vi "Read Message Type and Terminals.vi"(8 "error in":errorcluster, 11 "message ref in":refnum<k20>) -> (0 "error out":errorcluster, 2 "message type":T3, 3 "message ref out":refnum<k20>, 4 "Rx terminal":T1, 6 "Tx terminal":T1)   [LabVIEW 2020, in "MIL-STD 1553 Import.lvlib"]
uses:
  MIL-STD 1553 Import.lvlib
  Shared/Message Type.ctl
  Shared/Terminal Endpoint.ctl
  Shared/Address.ctl
  40e07135-e19e-4b22-895a-2c183958625d.vi
  487ea7c7-ffca-4428-88f2-a900c8ae7e8d.vi
  40e07135-e19e-4b22-895a-2c183958625d.vi/b1e6fcf8-dac1-42d2-b1fe-151afe06dbd4.vi
  487ea7c7-ffca-4428-88f2-a900c8ae7e8d.vi/b1e6fcf8-dac1-42d2-b1fe-151afe06dbd4.vi
  Constants.vi
  <vilib>/xml/Get Node Text Content.vi
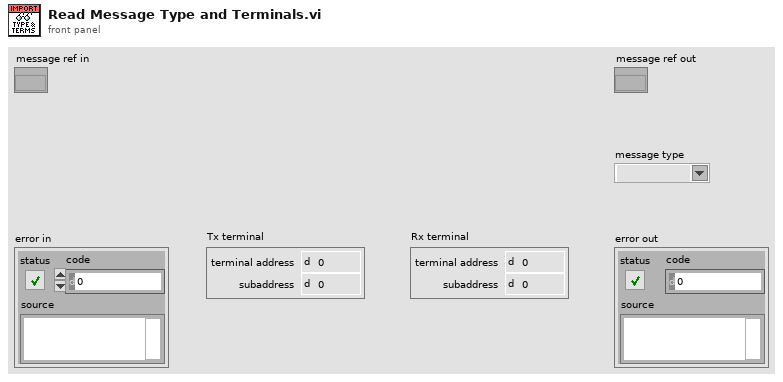
[diagram p1: front panel]
types:
  T1 = typedef "Terminal Endpoint.ctl" = cluster{"terminal address":T2, "subaddress":T2}
  T2 = typedef "Address.ctl" = u16
  T3 = typedef "Message Type.ctl" = string
  T4 = cluster{"terminal address":bool, "subaddress":bool}
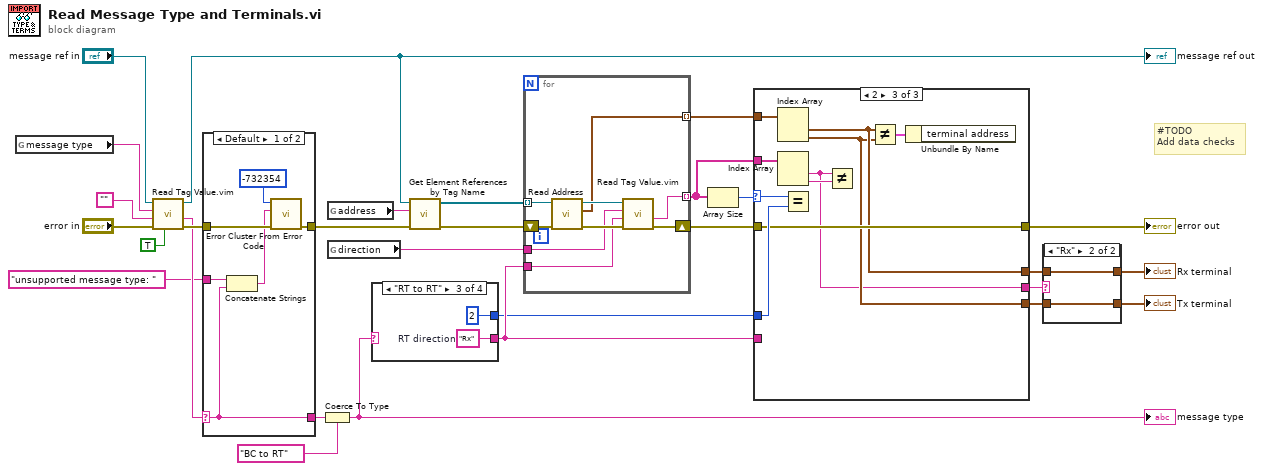
[diagram p0: block diagram]
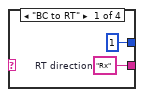
[diagram p3: hidden frame]
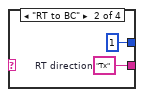
[diagram p4: hidden frame]
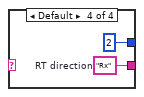
[diagram p5: hidden frame]
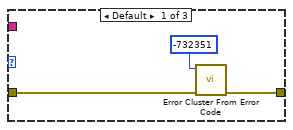
[diagram p6: hidden frame]
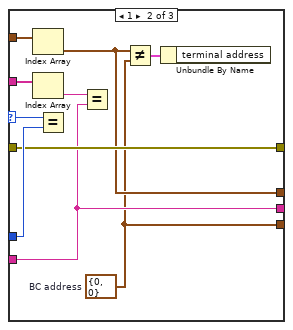
[diagram p7: hidden frame]
diagram:
  # "#TODO\nAdd data checks"
  n1 = global read "Constants.vi" "message type"() -> (w29:string)
  n2 = call "Read Tag Value.vim"("required (F)"=TRUE, "error in"="error in", "default"="", "tag name"=w29, "node in"="message ref in") -> ("error out"=w23:errorcluster, "value"=w22:string, "node out"=w19:refnum<k20>)  [unwired: 4 in]
  "message ref out" <- w19
  n3 = case shown="Default" w22 {
    selector: w22 -> [w31 w36]
    tunnel: [w34 w37] -> w21
    tunnel: w23 -> [w35 w37]
    tunnel: [w31 w36] -> w25
    tunnel: "unsupported message type: " -> [w32 _]
    frame Default {
      n4 = Concatenate Strings(w32, w31) -> (w30:string)
      n5 = call <vilib>:"Error Cluster From Error Code.vi"("error in (no error)"=w35, "error message (\"\")"=w30, "error code (0)"=-732354) -> ("error out"=w34:errorcluster)  [unwired: 6 in]
    }
    frame "BC to RT", "MC", "RT to BC", "RT to RT" {
    }
  }
  n6 = Coerce To Type(0:w25, 1:T3 "BC to RT" ("message type")) -> (2:w7:T3)
  "message type" <- w7
  n7 = global read "Constants.vi" "address"() -> (w20:string)
  n8 = global read "Constants.vi" "direction"() -> (w16:string)
  n9 = case shown="\"RT to RT\"" w7 {
    tunnel: [w39 w41 w43 w45] -> w9
    tunnel: [1 1 2 2] -> w8
    frame "BC to RT" {
      w39 = "Rx"  # RT direction
    }
    frame "RT to BC" {
      w41 = "Tx"  # RT direction
    }
    frame "RT to RT" {
      w43 = "Rx"  # RT direction
    }
    frame Default {
      w45 = "Rx"  # RT direction
    }
  }
  n10 = call "Get Element References by Tag Name.vi"("error in"=w21, "tag name"=w20, "node in"=w19) -> ("error out"=w18:errorcluster, "array of elements"=w17:refnum<k20>[])  [unwired: 7 in]
  n11 = for {
    shift-right: [w52] -> w15
    shift-left: w18 -> [w54]
    tunnel: w17 -> [w51] mode=indexing
    tunnel: w16 -> [w49]
    tunnel: w9 -> [w48]
    tunnel: [w47] -> w11 mode=indexing
    tunnel: [w46] -> w10 mode=indexing
    n12 = call "Read Address.vi"("error in"=w54, "address ref in"=w51) -> ("error out"=w53:errorcluster, "terminal"=w46:T1, "address ref out"=w50:refnum<k20>)  [unwired: 7 in]
    n13 = call "Read Tag Value.vim"("error in"=w53, "default"=w48, "tag name"=w49, "node in"=w50) -> ("error out"=w52:errorcluster, "value"=w47:string)  [unwired: 5 in, 1 out]
  }
  n14 = Array Size(array=w11) -> (size(s)=w12:i32)
  n15 = case shown="2" w12 {
    selector: w12 -> [_ w63 w74]
    tunnel: w15 -> [w56 w61 w71]
    tunnel: [w55 w61 w71] -> w14
    tunnel: w11 -> [_ w67 w77]
    tunnel: w10 -> [_ w66 w76]
    tunnel: w9 -> [_ w60 _]
    tunnel: w8 -> [_ w62 w73]
    tunnel: [_ w59 w70] -> w4
    tunnel: [_ w58 w69] -> w3
    tunnel: [_ w60 w68] -> w5
    frame Default {
      n16 = call <vilib>:"Error Cluster From Error Code.vi"("error in (no error)"=w56, "error code (0)"=-732351) -> ("error out"=w55:errorcluster)  [unwired: 7 in]
    }
    frame 1 {
      w58 = T1 {"terminal address"=0, "subaddress"=0}  # BC address
      n17 = Index Array(array=w66) -> (element=w59:T1)  [unwired: 1 in]
      n18 = Index Array(array=w67) -> (element=w64:string)  [unwired: 1 in]
      n19 = Equal?(x=w63, y=w62) -> ()  [unwired: 1 out]
      n20 = Equal?(x=w64, y=w60) -> ()  [unwired: 1 out]
      n21 = Not Equal?(x=w59, y=w58) -> (x != y?=w65:T4)
      n22 = Unbundle By Name(w65) -> ()  [unwired: 1 out]
    }
    frame 2 {
      n23 = Index Array(array=w76) -> (element #1=w70:T1, element #2=w69:T1)  [unwired: 2 in]
      n24 = Index Array(array=w77) -> (element #1=w68:string, element #2=w72:string)  [unwired: 2 in]
      n25 = Equal?(x=w74, y=w73) -> ()  [unwired: 1 out]
      n26 = Not Equal?(x=w68, y=w72) -> ()  [unwired: 1 out]
      n27 = Not Equal?(x=w70, y=w69) -> (x != y?=w75:T4)
      n28 = Unbundle By Name(w75) -> ()  [unwired: 1 out]
    }
  }
  "error out" <- w14
  n29 = case shown="\"Rx\"" w5 {
    tunnel: w4 -> [w78 w81]
    tunnel: [w79 w81] -> w2
    tunnel: [w78 w80] -> w1
    tunnel: w3 -> [w79 w80]
    frame Default {
    }
    frame "Rx" {
    }
  }
  "Rx terminal" <- w2
  "Tx terminal" <- w1
